vi "VariablesToString_old.vi"(1 "Value":dbl format="%.2f", 2 "Key Word":string="key wod") -> (0 "Concatenated String":string="key wod=;\r\n")   [LabVIEW 2011]
panel:
  in  "Format String":string="%f"
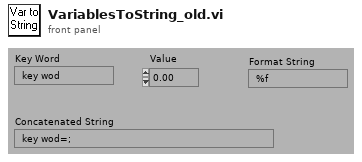
[diagram p1: front panel]
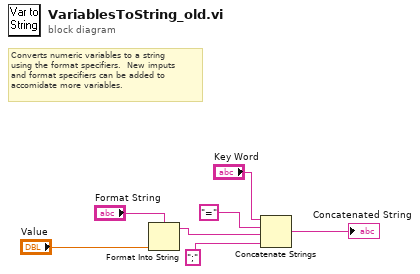
[diagram p0: block diagram]
diagram:
  # "Converts numeric variables to a string\nusing the format specifiers.  New imputs\nand format specifiers can be added to\naccomidate more variables."
  n1 = Format Into String(format string="Format String", "Value") -> (resulting string=w2:string)  [unwired: 2 in, 1 out]
  n2 = Concatenate Strings("Key Word", "=" ("Substring"), w2, ";" ("Substring")) -> (→"Concatenated String":string)
